vi "Save to EXCEL.vi"(8 "error in (no error)":errorcluster caption="错误输入（无错误）", 10 "text data":string[][](array[string])) -> (0 "error out":errorcluster caption="错误输出")   [LabVIEW 2018]
uses:
  <vilib>/addons/_office/_exclsub.llb/font.ctl
  <vilib>/addons/_office/excel.llb/Excel Easy Table (str).vi
  <vilib>/Utility/NIReport.llb/NI_report.lvclass
  <vilib>/addons/_office/NI_ReportGenerationToolkit.lvlib
  <vilib>/Utility/NIReport.llb/Excel/NI_Excel.lvclass
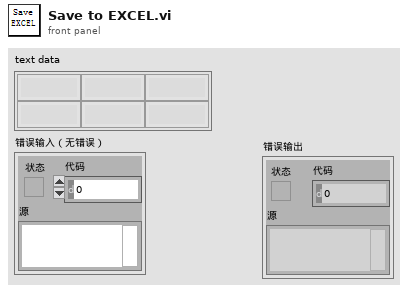
[diagram p1: front panel]
types:
  T1 = typedef "NI_ReportGenerationToolkit.lvlib/font.ctl" = cluster{"font name":string, "font size":dbl, "bold":u16, "italic":u16, "underline":u16, "strike through":u16, "font color":u32}
  T2 = enum16{"Standard Report", "HTML", "Word", "Excel"}
  T3 = enum16{"maximized", "minimized", "normal", "no change"}
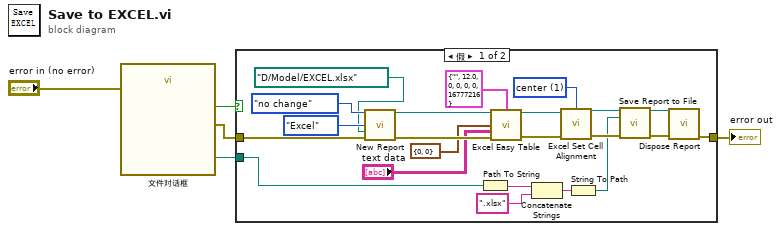
[diagram p0: block diagram]
diagram:
  n1 = call "文件对话框"("error in"="error in (no error)") -> ("selected path"=w1:path, "cancelled"=w3:bool, "error out"=w2:errorcluster)  [unwired: 11 in, 1 out]
  n2 = case shown="假" w3 {
    tunnel: [w17 w28] -> w5
    tunnel: w2 -> [w16 w28]
    tunnel: w1 -> [w8 _]
    frame False {
      w24 = 1 items=["left", "center", "right"] ("horizontal alignment (left)")
      n3 = call <vilib>:"New Report.vi"("window state (normal)"=T3."no change", "report type"=T2."Excel", "template (empty)"=path "D:/Model/EXCEL.xlsx", "error in (no error)"=w16) -> ("report out"=w20:refnum<class "NI_report.lvclass">, "error out"=w21:errorcluster)  [unwired: 10 in]
      n4 = Path To String(path=w8) -> (string=w11:string)
      n5 = call-poly <vilib>:"Excel Easy Table.vi"("report in"=w20, "font"=T1 {"font name"="", "font size"=12.0, "bold"=0, "italic"=0, "underline"=0, "strike through"=0, "font color"=16777216}, "start (0, 0)"=cluster{"row":i32, "column":i32} {"row"=0, "column"=0}, "text data"="text data", "error in (no error)"=w21) -> ("report out"=w22:refnum<class "NI_report.lvclass">, "error out"=w23:errorcluster)  [unwired: 6 in, 3 out]
      n6 = Concatenate Strings(w11, ".xlsx" ("字符串")) -> (w9:string)
      n7 = call <vilib>:"Excel Set Cell Alignment.vi"("report in"=w22, "horizontal alignment (left)"=w24, "error in (no error)"=w23) -> ("report out"=w12:refnum<class "NI_report.lvclass">, "error out"=w15:errorcluster)  [unwired: 11 in]
      n8 = String To Path(string=w9) -> (path=w7:path)
      n9 = call-dynamic "Save Report to File.vi"("report in"=w12, "report file path"=w7, "error in (no error)"=w15) -> ("report out"=w13:refnum<class "NI_report.lvclass">, "error out"=w14:errorcluster)  [unwired: 11 in]
      n10 = call-dynamic "Dispose Report.vi"("report in"=w13, "error in (no error)"=w14) -> ("error out"=w17:errorcluster)  [unwired: 13 in]
    }
    frame True {
    }
  }
  "error out" <- w5
